vi "FileLauncher.vi"() -> ()   [LabVIEW 2013]
panel:
  out "Files":string[](array[string])
  in  "Load file":path
  in  "Stop":bool=TRUE
  in  "Files_temp":string[](array[string])
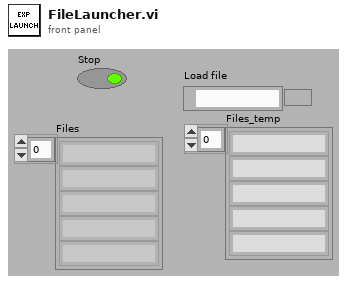
[diagram p1: front panel]
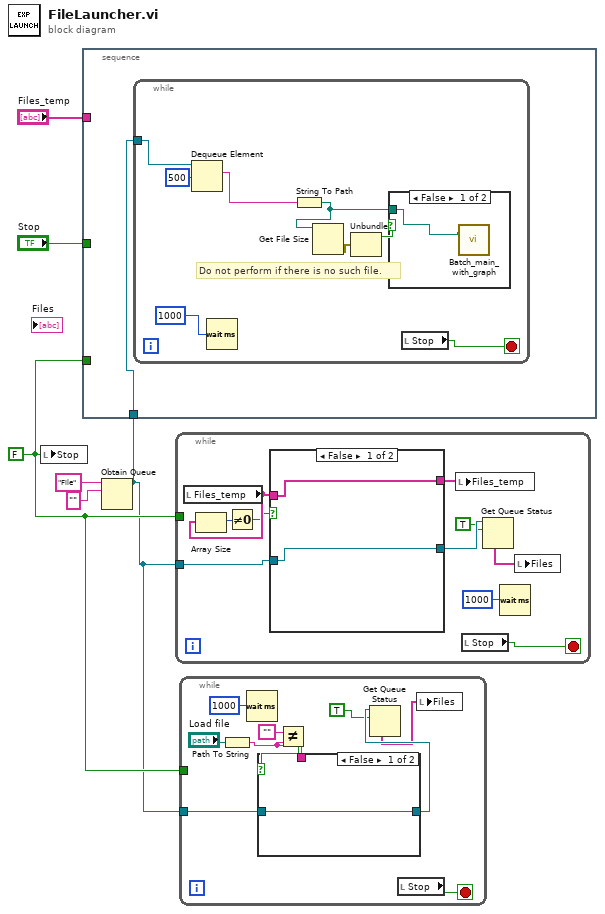
[diagram p0: block diagram]
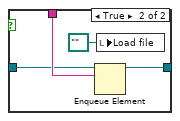
[diagram p2: hidden frame]
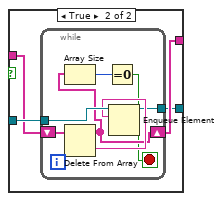
[diagram p3: hidden frame]
diagram:
  w4 = FALSE
  n1 = local write "Stop"(w4) -> ()
  n2 = Obtain Queue(name (unnamed)="File", element data type="") -> (queue out=w1:refnum<queue>)  [unwired: 3 in, 2 out]
  n3 = stacked-sequence {
    tunnel: "Stop" -> [_]
    tunnel: "Files_temp" -> [_]
    tunnel: w4 -> [_]
    tunnel: w1 -> [w7]
    frame #0 {
      n4 = while {
        tunnel: w7 -> [w10]
        stop <- w14 stop-if-true
        # "Do not perform if there is no such file."
        n5 = Dequeue Element(queue=w10, timeout in ms (-1)=500) -> (element=w9:string)  [unwired: 1 in, 3 out]
        n6 = Wait (ms)(milliseconds to wait=1000) -> ()  [unwired: 1 out]
        n7 = String To Path(string=w9) -> (path=w11:path)
        n8 = Get File Size(file=w11) -> (0:w13:errorcluster)  [unwired: 1 in, 2 out]
        n9 = Unbundle(w13) -> ("status"=w12:bool)  [unwired: 2 out]
        n10 = case shown="False" w12 {
          tunnel: w11 -> [w16 _]
          frame False {
            n11 = call "Batch_main_with_graph.vi"("ExpFilePath"=w16) -> ()  [unwired: 2 in]
          }
          frame True {
          }
        }
        n12 = local read "Stop"() -> (w14:bool)
      }
    }
  }
  n13 = while {
    tunnel: w4 -> [_]
    tunnel: w1 -> [w20]
    stop <- w21 stop-if-true
    n14 = local read "Files_temp"() -> (w23:string[])
    n15 = Array Size(array=w23) -> (size(s)=w24:i32)
    n16 = Not Equal To 0?(x=w24) -> (x != 0?=w22:bool)
    n17 = case shown="False" w22 {
      tunnel: w23 -> [w28 w31]
      tunnel: [w28 w30] -> w26
      tunnel: w20 -> [w27 w32]
      tunnel: [w27 w29] -> w19
      frame False {
      }
      frame True {
        n18 = while {
          tunnel: w32 -> [w39]
          shift-right: [w36] -> w30
          shift-left: w31 -> [w38]
          tunnel: [w33] -> w29
          stop <- w34 stop-if-true
          n19 = Delete From Array(array=w38) -> (deleted portion=w37:string, array with subset deleted=w36:string[])  [unwired: 2 in]
          n20 = Array Size(array=w36) -> (size(s)=w35:i32)
          n21 = Equal To 0?(x=w35) -> (x = 0?=w34:bool)
          n22 = Enqueue Element(queue=w39, element=w37) -> (queue out=w33:refnum<queue>)  [unwired: 2 in, 2 out]
        }
      }
    }
    n23 = local write "Files_temp"(w26) -> ()
    n24 = local read "Stop"() -> (w21:bool)
    n25 = Get Queue Status(queue=w19, return elements? (F)=TRUE) -> (elements=w18:string[])  [unwired: 1 in, 7 out]
    n26 = Wait (ms)(milliseconds to wait=1000) -> ()  [unwired: 1 out]
    n27 = local write "Files"(w18) -> ()
  }
  n28 = while {
    tunnel: w4 -> [_]
    tunnel: w1 -> [w43]
    stop <- w48 stop-if-true
    n29 = Path To String(path="Load file") -> (string=w45:string)
    n30 = Wait (ms)(milliseconds to wait=1000) -> ()  [unwired: 1 out]
    n31 = Not Equal?(x="", y=w45) -> (x != y?=w44:bool)
    n32 = case shown="False" w44 {
      tunnel: w45 -> [_ w53]
      tunnel: w43 -> [w50 w52]
      tunnel: [w50 w51] -> w42
      frame False {
      }
      frame True {
        n33 = Enqueue Element(queue=w52, element=w53) -> (queue out=w51:refnum<queue>)  [unwired: 2 in, 2 out]
        n34 = local write "Load file"(path "") -> ()
      }
    }
    n35 = Get Queue Status(queue=w42, return elements? (F)=TRUE) -> (elements=w41:string[])  [unwired: 1 in, 7 out]
    n36 = local read "Stop"() -> (w48:bool)
    n37 = local write "Files"(w41) -> ()
  }
